vi "Configure File Observers.vi"(8 "error in":errorcluster, 11 "tCRD in":refnum<class "tCRD.lvclass">) -> (0 "error out":errorcluster, 3 "tCRD out":refnum<class "tCRD.lvclass">)   [LabVIEW 2015, in "tCRD.lvclass"]
doc: "Configure file observers for file saving."
uses:
  tCRD.lvclass
  Data Subj/tCRDS Subj.lvclass
  Reusable/Observer/Data Subject.lvclass
  File Observer/Tim File Observer.lvclass
  <vilib>/Utility/config.llb/NI_LVConfig.lvlib
  <vilib>/Utility/config.llb/Read Key (Boolean).vi
  <vilib>/Utility/config.llb/Read Key (I32).vi
  <vilib>/Utility/config.llb/Read Key (Path).vi
  <vilib>/Utility/config.llb/Read Key (String).vi
  Reusable/File IO/Class/File Observer.lvclass
  Reusable/Session APIs/File Access/Config Data/Config Data.lvclass
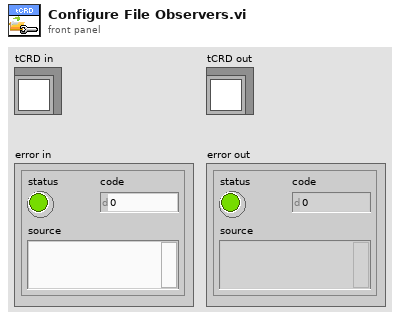
[diagram p1: front panel]
types:
  T1 = typedef "Session - Root.lvclass/Session Handle.ctl" = refnum<data-value>
  T2 = typedef "NI_LVConfig.lvlib/Config Data RefNum.ctl" = refnum<k1>
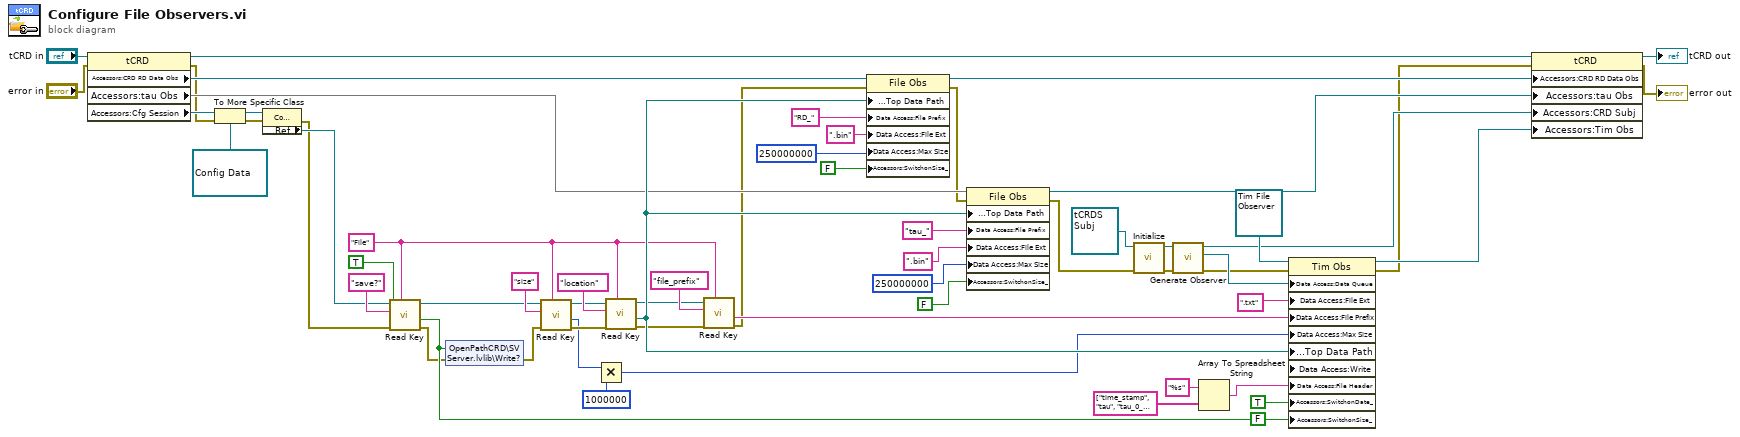
[diagram p0: block diagram]
diagram:
  w45 = "File" ("section")
  n1 = property class="tCRD"(reference="tCRD in", error in="error in") -> (reference out=w8:refnum<class "tCRD.lvclass">, error out=w18:errorcluster, "Accessors:CRD RD Data Obs"=w58:refnum<class "File Observer.lvclass">, "Accessors:tau Obs"=w59, "Accessors:Cfg Session"=w22:T1)
  n2 = To More Specific Class(target class=refnum<data-value> refnum, reference=w22, error in=w18) -> (specific class reference=w21:refnum<data-value>, error out=w17:errorcluster)
  n3 = property class="Config Data"(reference=w21, error in=w17) -> (error out=w15:errorcluster, "Accessors:Ref"=w16:T2)  [unwired: 1 out]
  n4 = call-poly <vilib>:"Read Key.vi"("section"=w45, "error in (no error)"=w15, "default value"=TRUE, "key"="save?", "refnum"=w16) -> ("error out"=w14:errorcluster, "value"=w33:bool, "refnum out"=w35:T2)  [unwired: 3 in, 1 out]
  n5 = shared-variable "OpenPathCRD\\SV Server.lvlib\\Write?"(w33, error in=w14) -> (error out=w13:errorcluster)
  n6 = call-poly <vilib>:"Read Key.vi"("section"=w45, "error in (no error)"=w13, "key"="size", "refnum"=w35) -> ("error out"=w41:errorcluster, "value"=w37:i32, "refnum out"=w40:T2)  [unwired: 4 in, 1 out]
  n7 = Multiply(x=w37, y=1000000 ("x")) -> (x*y=w39:i32)
  n8 = call-poly <vilib>:"Read Key.vi"("section"=w45, "error in (no error)"=w41, "key"="location", "refnum"=w40) -> ("error out"=w44:errorcluster, "value"=w60:path, "refnum out"=w43:T2)  [unwired: 4 in, 1 out]
  n9 = call-poly <vilib>:"Read Key.vi"("section"=w45, "error in (no error)"=w44, "key"="file_prefix", "refnum"=w43) -> ("error out"=w12:errorcluster, "value"=w47:string)  [unwired: 4 in, 2 out]
  n10 = property class="File Obs"(reference=w58, error in=w12, "Data Access:Top Data Path"=w60, "Data Access:File Prefix"="RD_" ("File Prefix"), "Data Access:File Ext"=".bin" ("File Prefix"), "Data Access:Max Size"=i64 250000000 ("Max Size"), "Accessors:SwitchonSize_"=FALSE ("SwitchonSize_")) -> (reference out=w7:refnum<class "File Observer.lvclass">, error out=w11:errorcluster)
  n11 = property class="File Obs"(reference=w59, error in=w11, "Data Access:Top Data Path"=w60, "Data Access:File Prefix"="tau_" ("File Prefix"), "Data Access:File Ext"=".bin" ("File Prefix"), "Data Access:Max Size"=i64 250000000 ("Max Size"), "Accessors:SwitchonSize_"=FALSE ("SwitchonSize_")) -> (reference out=w6:refnum<class "File Observer.lvclass">, error out=w10:errorcluster)
  n12 = call-dynamic "Initialize.vi"("error in"=w10, "tCRDS Subj in"=refnum<class "tCRDS Subj.lvclass"> refnum ("tCRDS Subj.lvclass")) -> ("error out"=w24:errorcluster, "tCRDS Subj out"=w23:refnum<class "tCRDS Subj.lvclass">)  [unwired: 7 in, 1 out]
  n13 = call "Generate Observer.vi"("error in"=w24, "Data Subject in"=w23) -> ("error out"=w9:errorcluster, "Observer"=w25:refnum<queue>, "Data Subject out"=w5:refnum<class "tCRDS Subj.lvclass">)  [unwired: 7 in]
  n14 = Array To Spreadsheet String(array=string[] ["time_stamp", "tau", "tau_0_corr", "ext", "ext_corr", "std_dev_tau", "e_tau", "tau_corr", "tau_0", "max_amplitude", "RH_vaisala", "T_vaisala", "V_anemom", "zero", "latittude", "north_south", "longitude", "east_wet", "GPS_qual", "num_satellites", "MSL_altitude", "pressure", "T_external", "RH_external", "Td_external", "true_wind_dir", "magnetic_wind_dir", "wind_speed", "Palicat", "Qalicat", "Q0alicat", "Talicat", "Qspalicat", "RH_Rotronic", "T_Rotronic"], 3:"%s" ("format string")) -> (spreadsheet string=w29:string)  [unwired: 1 in]
  n15 = property class="Tim Obs"(reference=refnum<class "Tim File Observer.lvclass"> refnum ("Tim Obs"), error in=w9, "Data Access:Data Queue"=w25, "Data Access:File Ext"=".txt" ("File Ext"), "Data Access:File Prefix"=w47, "Data Access:Max Size"=w39, "Data Access:Top Data Path"=w60, "Data Access:Write"=w33, "Data Access:File Header"=w29, "Accessors:SwitchonDate_"=TRUE ("SwitchonDate_"), "Accessors:SwitchonSize_"=FALSE ("SwitchonSize_")) -> (reference out=w4:refnum<class "Tim File Observer.lvclass">, error out=w3:errorcluster)
  n16 = property class="tCRD"(reference=w8, error in=w3, "Accessors:CRD RD Data Obs"=w7, "Accessors:tau Obs"=w6, "Accessors:CRD Subj"=w5, "Accessors:Tim Obs"=w4) -> (reference out=→"tCRD out":refnum<class "tCRD.lvclass">, error out=→"error out":errorcluster)
